vi "MakeLegend.vi"(11 "WaveNum":u32) -> (3 "Legend Out":picture caption="LegendOut")   [LabVIEW 2012, in "WaveGraphX.xctl"]
uses:
  WaveGraphX.xctl
panel:
  in  "plot info":T1(array[cluster])=[{"plot name"="Wave 01", "plot color"=16711680, "fill?(F)"=FALSE}, {"plot name"="Wave 02", "plot color"=14450432, "fill?(F)"=FALSE}, {"plot name"="Wave 03", "plot color"=32639, "fill?(F)"=FALSE}, {"plot name"="Wave 04", "plot color"=16860, "fill?(F)"=FALSE}]
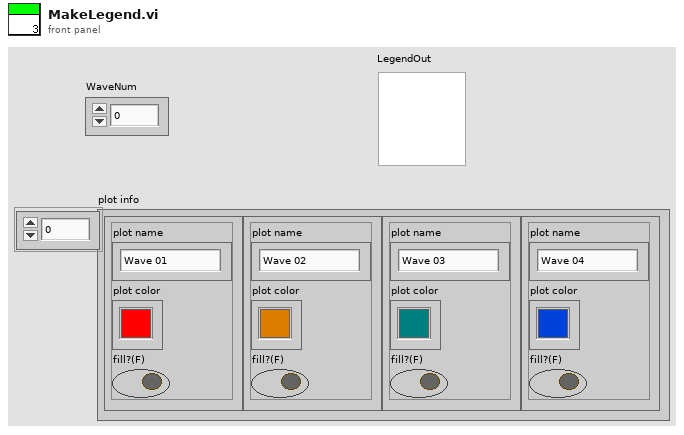
[diagram p1: front panel]
types:
  T1 = cluster{"plot name":string, "plot color":u32, "fill?(F)":bool}[]
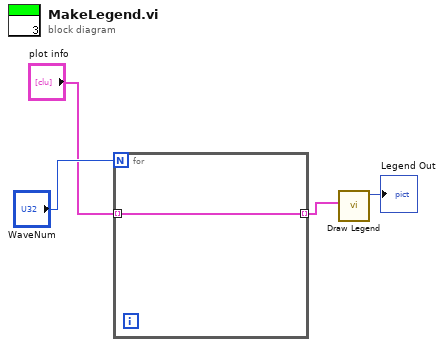
[diagram p0: block diagram]
diagram:
  n1 = for {
    N: "WaveNum" -> [_]
    tunnel: "plot info" -> [w5] mode=indexing
    tunnel: [w5] -> w1 mode=indexing
  }
  n2 = call <vilib>:"Draw Legend.vi"("plot info"=w1) -> ("new picture"=→"Legend Out":picture)  [unwired: 10 in]
